vi "ADCP_Processed_Bytes_To_ES_Packet.vi"(8 "error in (no error)":errorcluster, 10 "Processed Packet Bytes":u8[](array[numeric]), 11 "ADCP In":refnum<class "ADCP.lvclass">) -> (0 "error out":errorcluster, 2 "ES Packet":T1, 3 "ADCP Out":refnum<class "ADCP.lvclass">)   [LabVIEW 2017, in "ADCP.lvclass"]
uses:
  ADCP.lvclass
  ADCP.lvclass/ADCP.ctl
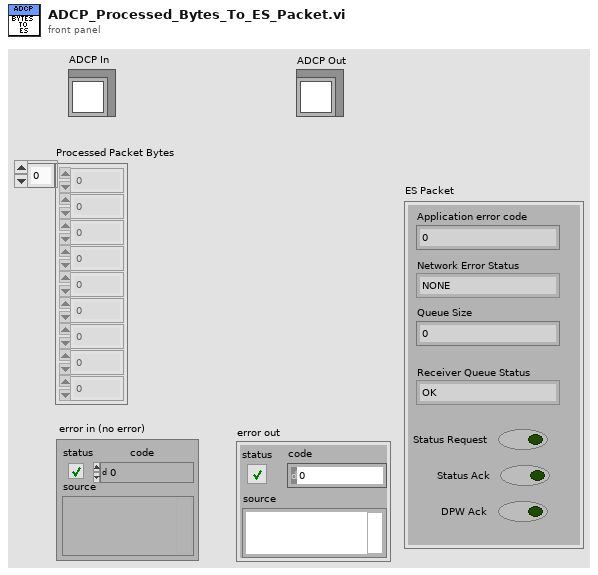
[diagram p1: front panel]
types:
  T1 = cluster{"Application error code":u16, "Network Error Status":enum16{"NONE", "CONNECTION_ALREADY_OPEN", "CONNECTION_ALREADY_CLOSED", "INVALID_FRAME_REQUEST"}, "Queue Size":u16, "Receiver Queue Status":enum16{"OK", "EMPTY", "FULL"}, "Status Request":bool, "Status Ack":bool, "DPW Ack":bool}
  T2 = enum16{"Data", "Connection Management", "Remote Request", "Error and status", "INVALID"}
  T3 = cluster{"Application error code":u16, "Network Error Status":enum16{"NONE", "CONNECTION_ALREADY_OPEN", "CONNECTION_ALREADY_CLOSED", "INVALID_FRAME_REQUEST"}, "Queue Size":u16, "Receiver Queue Status":enum16{"OK", "EMPTY", "FULL"}, "Status Request":bool, "Status Ack":bool, "WDP Ack":bool}
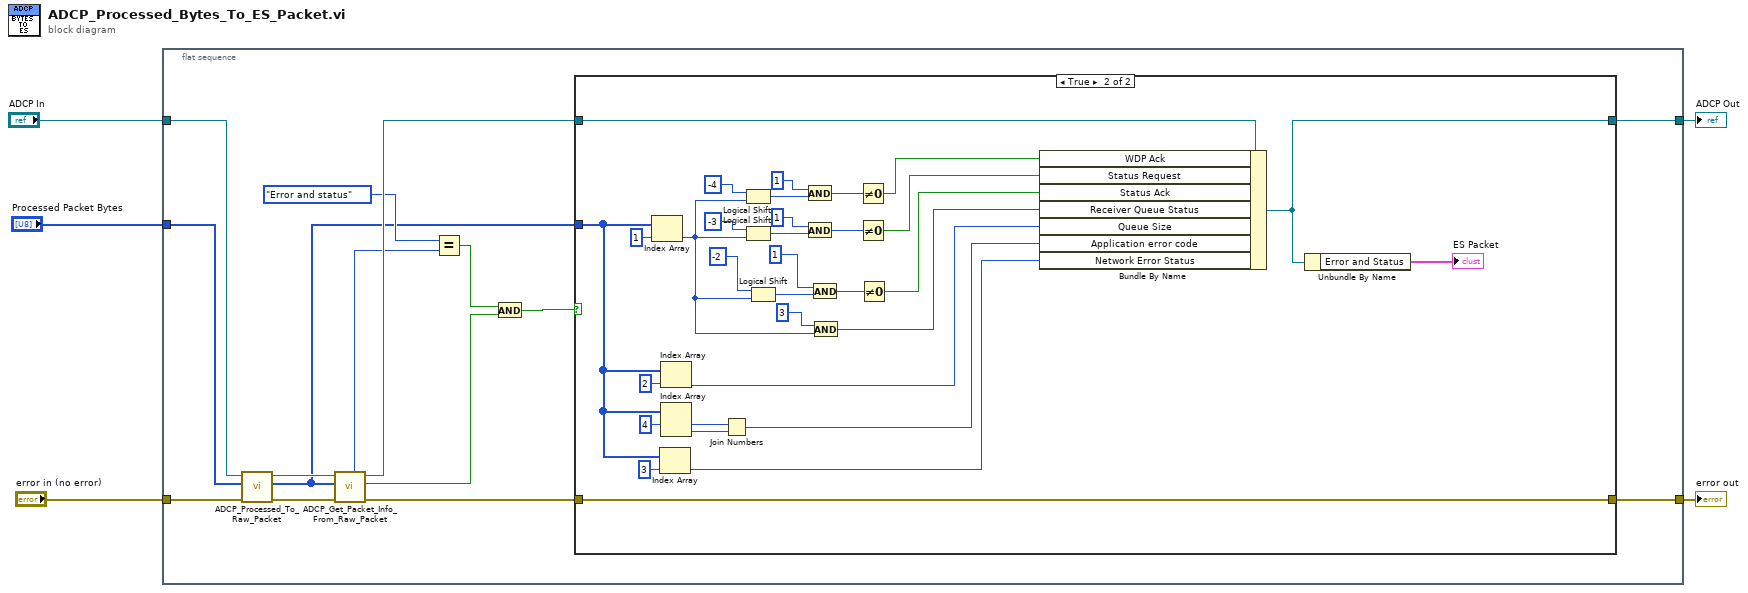
[diagram p0: block diagram]
diagram:
  n1 = flat-sequence {
    tunnel: "ADCP In" -> [w17]
    tunnel: "Processed Packet Bytes" -> [w18]
    tunnel: "error in (no error)" -> [w19]
    tunnel: [w20] -> w2
    tunnel: [w7] -> w1
    frame #0 {
      n2 = call "ADCP_Processed_To_Raw_Packet.vi"("error in (no error)"=w19, "Processed Packet"=w18, "ADCP in"=w17) -> ("error out"=w16:errorcluster, "Raw Packet"=w6:u8[], "ADCP out"=w15:refnum<class "ADCP.lvclass">)  [unwired: 6 in]
      n3 = call "ADCP_Get_Packet_Info_From_Raw_Packet.vi"("error in (no error)"=w16, "Raw Packet"=w6, "ADCP in"=w15) -> ("error out"=w11:errorcluster, "Checksum Valid ?"=w8:bool, "ADCP out"=w14:refnum<class "ADCP.lvclass">, "Packet Type"=w13:T2)  [unwired: 2 in, 3 out]
      n4 = Equal?(x=T2."Error and status", y=w13) -> (x = y?=w10:bool)
      n5 = And(x=w10, y=w8) -> (x .and. y?=w9:bool)
      n6 = case shown="True" w9 {
        tunnel: [w22 w30] -> w20
        tunnel: w14 -> [w22 w54]
        tunnel: w11 -> [w21 w31]
        tunnel: [w21 w31] -> w7
        tunnel: w6 -> [_ w34]
        frame False {
        }
        frame True {
          n7 = Index Array(array=w34, index=1) -> (element=w24:u8)
          n8 = Index Array(array=w34, index=3) -> (element=w32:u8)
          n9 = Index Array(array=w34, index=2) -> (element=w39:u8)
          n10 = Index Array(array=w34, index #1=4 ("index")) -> (element #1=w37:u8, element #2=w36:u8)  [unwired: 1 in]
          n11 = Join Numbers(hi=w37, lo=w36) -> ((hi.lo)=w35:u16)
          n12 = Logical Shift(y=i16 -4, x=w24) -> (x << y=w27:u8)
          n13 = Logical Shift(y=i16 -3, x=w24) -> (x << y=w52:u8)
          n14 = Logical Shift(y=i16 -2, x=w24) -> (x << y=w49:u8)
          n15 = And(x=u8 1, y=w27) -> (x .and. y?=w25:u8)
          n16 = And(x=u8 1, y=w52) -> (x .and. y?=w46:u8)
          n17 = And(x=u8 1, y=w49) -> (x .and. y?=w45:u8)
          n18 = And(x=u8 3, y=w24) -> (x .and. y?=w42:u8)
          n19 = Not Equal To 0?(x=w25) -> (x != 0?=w23:bool)
          n20 = Not Equal To 0?(x=w46) -> (x != 0?=w44:bool)
          n21 = Not Equal To 0?(x=w45) -> (x != 0?=w43:bool)
          n22 = Bundle By Name(cluster=w54, "WDP Ack"=w23, "Status Request"=w44, "Status Ack"=w43, "Receiver Queue Status"=w42, "Queue Size"=w39, "Application error code"=w35, "Network Error Status"=w32) -> (w30:refnum<class "ADCP.lvclass">)
          n23 = Unbundle By Name(w30) -> ("Error and Status"=→"ES Packet":T3)
        }
      }
    }
  }
  "ADCP Out" <- w2
  "error out" <- w1
